vi "RSNRPZ Get Scope Measurements Pulse Levels.vi"(8 "error in (no error)":errorcluster, 10 "Channel (1)":i32=1, 11 "VISA session":refnum<visa-resource-name> caption="VISA resource name") -> (0 "error out":errorcluster, 1 "Top Level":dbl format="%^.3e", 3 "dup VISA session":refnum<visa-resource-name> caption="VISA resource name", 5 "Base Level":dbl format="%^.3e")   [LabVIEW 2010]
doc: "This VI returns the pulse top level and the pulse base level in watt. Both levels are calculated with the algorithm that was set with the rsnrpz_scope_meas_setMeasAlgorithm(...) VI.\n\nNote:\n1) This VI is only available for NRP-Z81.\n\nRemote-control command(s):\nSENS:TRAC:MEAS:POW:PULS:TOP?\nSENS:TRAC:MEAS:POW:PULS:BASE?"
uses:
  rsnrpz_32.dll
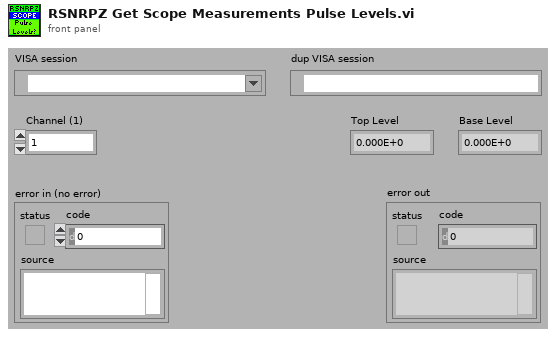
[diagram p1: front panel]
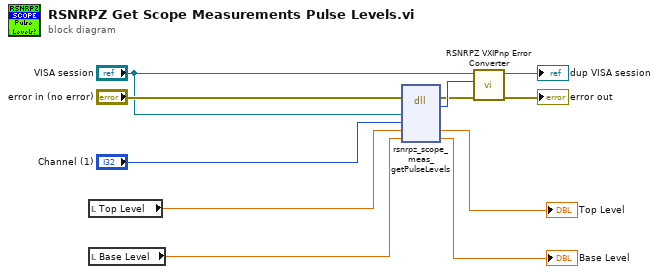
[diagram p0: block diagram]
diagram:
  n1 = local read "Top Level"() -> (w9:dbl)
  n2 = local read "Base Level"() -> (w7:dbl)
  n3 = dll-call lib="rsnrpz_32.dll" fn="rsnrpz_scope_meas_getPulseLevels"(error in="error in (no error)", "Instrument Handle"="VISA session", "Channel"="Channel (1)", "Top Level"=w9, "Base Level"=w7) -> (error out=w5:errorcluster, "Status"=w11:i32, "Top Level"=→"Top Level":dbl, "Base Level"=→"Base Level":dbl)  [unwired: 4 in, 1 out]
  n4 = call <instrlib>:"RSNRPZ VXIPnp Error Converter.vi"("error in"=w5, "VXIPnp error code"=w11, "VISA session"="VISA session") -> ("error out"=→"error out":errorcluster, "dup VISA session"=→"dup VISA session":refnum<visa-resource-name>)  [unwired: 7 in]
